vi "Configure Power Measurement Trigger.vi"(0 "VISA resource name":refnum<visa-resource-name>, 1 "Offset (0.1E-3)":dbl=0.0001 format="%^.3e", 2 "Slope (Rising)":i32(ring) items=["Rising", "Falling"], 5 "Instance (1)":i32=1 format="%.0g", 7 "Source (\"IF Power\")":string="IF Power", 9 "Threshold (-30.0)":dbl=-30.0 format="%^.3e", 11 "error in (no error)":errorcluster, 12 "Mode (Trigger Once)":i32(ring) items=["Trigger Once", "Retrigger Sweep", "Retrigger All", "Preselect"], 13 "Trigger Timeout (1.0)":dbl=1.0 format="%^.3e") -> (4 "VISA resource name out":refnum<visa-resource-name>, 15 "error out":errorcluster)   [LabVIEW 2015, in "Rohde&Schwarz CMXP GPRF.lvlib"]
doc: "Defines the trigger parameters.\n\nAttributes:\nRSCMXPGPRF_ATTR_POWER_MEASUREMENT_TRIGGER_SOURCE\nRSCMXPGPRF_ATTR_POWER_MEASUREMENT_TRIGGER_SLOPE\nRSCMXPGPRF_ATTR_POWER_MEASUREMENT_TRIGGER_THRESHOLD\nRSCMXPGPRF_ATTR_POWER_MEASUREMENT_TRIGGER_OFFSET\nRSCMXPGPRF_ATTR_POWER_MEASUREMENT_TRIGGER_MODE\nRSCMXPGPRF_ATTR_POWER_MEASUREMENT_TRIGGER_TIMEOUT\n\nRemote-control commands:\nTRIGger:GPRF:MEAS<i>:POWer:SOURce\nCONFigure:GPRF:MEAS<i>:POWer:TRIGger:SLOPe\nTRIGger:GPRF:MEAS<i>:POWer:THReshold\nTRIGger:GPRF:MEAS<i>:POWer:OFFSet\nTRIGger:GPRF:MEAS<i>:POWer:MODE\nTRIGger:GPRF:MEAS<i>:POWer:TOUT"
uses:
  <instrlib>/Rohde&Schwarz CMXP GPRF/Rohde&Schwarz CMXP GPRF.lvlib
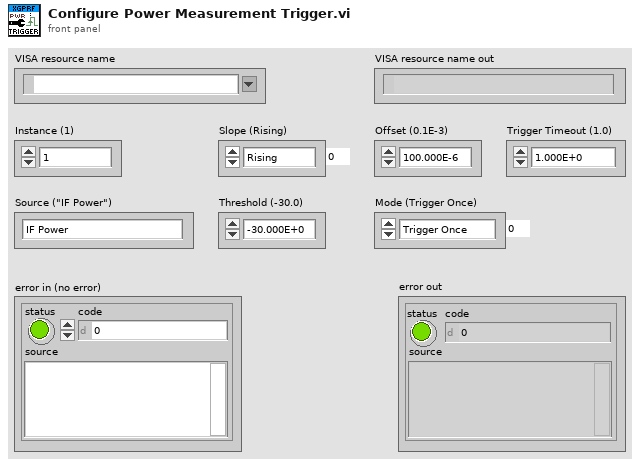
[diagram p1: front panel]
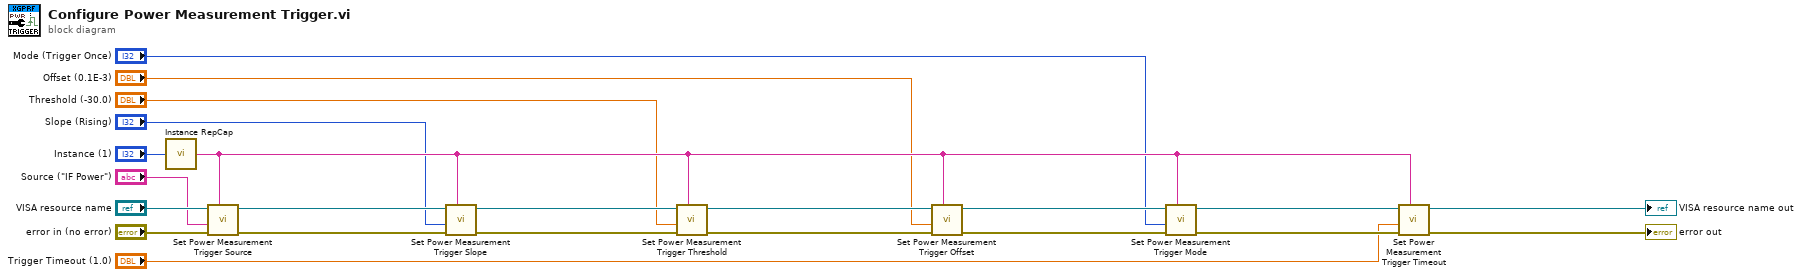
[diagram p0: block diagram]
diagram:
  n1 = call <instrlib>:"Instance RepCap.vi"("instance  in"="Instance (1)") -> ("instance out"=w7:string)
  n2 = call "Set Power Measurement Trigger Source"("Repeated Capabilities"=w7, "error in (no error)"="error in (no error)", "Power Measurement Trigger Source ()"="Source (\"IF Power\")", "instrument handle"="VISA resource name") -> ("error out"=w16:errorcluster, "instrument handle out"=w13:refnum<visa-resource-name>)  [unwired: 6 in]
  n3 = call "Set Power Measurement Trigger Slope"("Repeated Capabilities"=w7, "error in (no error)"=w16, "Power Measurement Trigger Slope (0 - Rising)"="Slope (Rising)", "instrument handle"=w13) -> ("error out"=w18:errorcluster, "instrument handle out"=w19:refnum<visa-resource-name>)  [unwired: 6 in]
  n4 = call "Set Power Measurement Trigger Threshold"("Repeated Capabilities"=w7, "error in (no error)"=w18, "Power Measurement Trigger Threshold (0.0)"="Threshold (-30.0)", "instrument handle"=w19) -> ("error out"=w21:errorcluster, "instrument handle out"=w20:refnum<visa-resource-name>)  [unwired: 6 in]
  n5 = call "Set Power Measurement Trigger Offset"("Repeated Capabilities"=w7, "error in (no error)"=w21, "Power Measurement Trigger Offset (0.0)"="Offset (0.1E-3)", "instrument handle"=w20) -> ("error out"=w22:errorcluster, "instrument handle out"=w17:refnum<visa-resource-name>)  [unwired: 6 in]
  n6 = call "Set Power Measurement Trigger Mode"("Repeated Capabilities"=w7, "error in (no error)"=w22, "Power Measurement Trigger Mode (0 - Trigger Once)"="Mode (Trigger Once)", "instrument handle"=w17) -> ("error out"=w11:errorcluster, "instrument handle out"=w8:refnum<visa-resource-name>)  [unwired: 6 in]
  n7 = call "Set Power Measurement Trigger Timeout"("Repeated Capabilities"=w7, "error in (no error)"=w11, "Power Measurement Trigger Timeout (0.0)"="Trigger Timeout (1.0)", "instrument handle"=w8) -> ("error out"=→"error out":errorcluster, "instrument handle out"=→"VISA resource name out":refnum<visa-resource-name>)  [unwired: 6 in]
